vi "Write LINX I2C Channel.vi"(8 "error in (no error)":errorcluster, 10 "LINX I2C Channel":u8=1, 11 "LINX-PCA9865 PWM in":refnum<class "LINX-PCA9865 PWM.lvclass">) -> (0 "error out":errorcluster, 3 "LINX-PCA9865 PWM out":refnum<class "LINX-PCA9865 PWM.lvclass">)   [LabVIEW 2019, in "LINX-PCA9865 PWM.lvclass"]
uses:
  LINX-PCA9865 PWM.lvclass
  LINX-PCA9865 PWM.lvclass/LINX-PCA9865 PWM.ctl
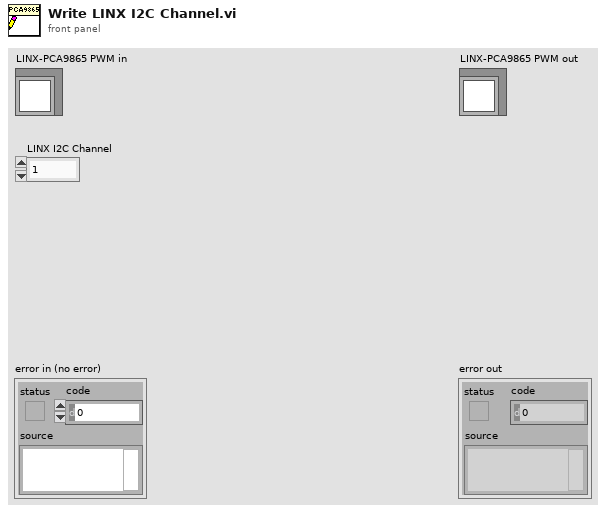
[diagram p1: front panel]
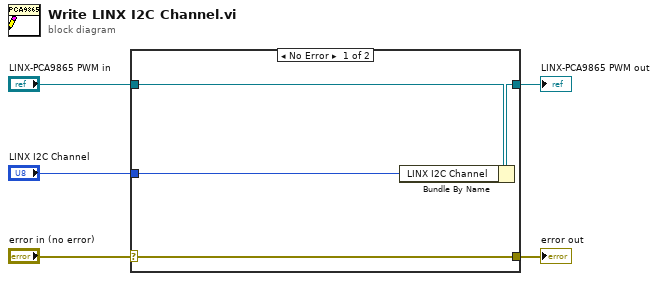
[diagram p0: block diagram]
diagram:
  n1 = case shown="No Error" "error in (no error)" {
    selector: "error in (no error)" -> [w9 w10]
    tunnel: [w9 w10] -> w4
    tunnel: [w7 w11] -> w2
    tunnel: "LINX-PCA9865 PWM in" -> [w8 w11]
    tunnel: "LINX I2C Channel" -> [w6 _]
    frame No Error {
      n2 = Bundle By Name(cluster=w8, "LINX I2C Channel"=w6) -> (w7:refnum<class "LINX-PCA9865 PWM.lvclass">)
    }
    frame Error {
    }
  }
  "error out" <- w4
  "LINX-PCA9865 PWM out" <- w2
